vi "Module_Configure_All SMUs_Manual.vi"(7 "Throw Settings":T4={"SMU Settings"={"CH"={"Voltage Limit"=1.0, "current limit"=0.01, "Voltage limit range"=6.0, "Current level"=0.01, "CH_RF1"="0", "Output Enabled"=TRUE}, "CH"={"Voltage Limit"=1.0, "current limit"=0.01, "Voltage limit range"=6.0, "Current level"=0.01, "CH_RF2"="1", "Output Enabled"=TRUE}, "CH"={"Voltage Limit"=1.0, "current limit"=0.01, "Voltage limit range"=6.0, "Current level"=0.01, "CH_RF3"="2", "Output Enabled"=TRUE}, "CH"={"Voltage Limit"=1.0, "current limit"=0.01, "Voltage limit range"=6.0, "Current level"=0.01, "CH_RF4"="3", "Output Enabled"=TRUE}}, "sense"=1008, "aperture time"=0.01666} {"aperture time" format="%.2p"; "sense" items=["Local"=1008, "Remote"=1009]; "SMU Settings"."CH"."Current level" format="%#.6p"; "SMU Settings"."CH"."Voltage limit range" format="%#.6p"; "SMU Settings"."CH"."current limit" format="%#.6p"; "SMU Settings"."CH"."Voltage Limit" format="%#.6p"; "SMU Settings"."CH"."Current level" format="%#.6p"; "SMU Settings"."CH"."Voltage limit range" format="%#.6p"; "SMU Settings"."CH"."current limit" format="%#.6p"; "SMU Settings"."CH"."Voltage Limit" format="%#.6p"; "SMU Settings"."CH"."Current level" format="%#.6p"; "SMU Settings"."CH"."Voltage limit range" format="%#.6p"; "SMU Settings"."CH"."current limit" format="%#.6p"; "SMU Settings"."CH"."Voltage Limit" format="%#.6p"; "SMU Settings"."CH"."Current level" format="%#.6p"; "SMU Settings"."CH"."Voltage limit range" format="%#.6p"; "SMU Settings"."CH"."current limit" format="%#.6p"; "SMU Settings"."CH"."Voltage Limit" format="%#.6p"}, 8 "Error In":errorcluster, 10 "DUT and Bridge SMU Settings":T5={"SMU Settings"={"CH"={"voltage level range"=6.0, "current limit"=0.1, "current limit range"=0.1, "voltage level "=1.2, "CH"="0", "Output Enabled"=FALSE}, "CH 2"={"voltage level range"=6.0, "current limit"=0.001, "current limit range"=0.001, "voltage level "=5.0, "CH"="1", "Output Enabled"=FALSE}, "CH 3"={"voltage level range"=6.0, "current limit"=0.001, "current limit range"=0.001, "voltage level "=-5.0, "CH"="2", "Output Enabled"=FALSE}, "CH 4"={"voltage level range"=6.0, "current limit"=0.01, "current limit range"=0.01, "voltage level "=1.8, "CH"="3", "Output Enabled"=FALSE}}, "sense"=1008, "aperture time"=0.01666} {"aperture time" format="%.2p"; "sense" items=["Local"=1008, "Remote"=1009]; "SMU Settings"."CH 4"."voltage level" format="%#.6p"; "SMU Settings"."CH 4"."current limit range" format="%#.6p"; "SMU Settings"."CH 4"."current limit" format="%#.6p"; "SMU Settings"."CH 4"."voltage level range" format="%#.6p"; "SMU Settings"."CH 3"."voltage level" format="%#.6p"; "SMU Settings"."CH 3"."current limit range" format="%#.6p"; "SMU Settings"."CH 3"."current limit" format="%#.6p"; "SMU Settings"."CH 3"."voltage level range" format="%#.6p"; "SMU Settings"."CH 2"."voltage level" format="%#.6p"; "SMU Settings"."CH 2"."current limit range" format="%#.6p"; "SMU Settings"."CH 2"."current limit" format="%#.6p"; "SMU Settings"."CH 2"."voltage level range" format="%#.6p"; "SMU Settings"."CH"."voltage level" format="%#.6p"; "SMU Settings"."CH"."current limit range" format="%#.6p"; "SMU Settings"."CH"."current limit" format="%#.6p"; "SMU Settings"."CH"."voltage level range" format="%#.6p"}, 11 "Instrument_Visas":T1) -> (0 "Error Out":errorcluster, 2 "DUR_4_CH_SMU":T3(array[cluster]) {"sense 2" items=["Local"=1008, "Remote"=1009]}, 3 "Throw_4_CH_SMU":T3(array[cluster]) {"sense 2" items=["Local"=1008, "Remote"=1009]})   [LabVIEW 2013]
uses:
  <instrlib>/niDCPower/nidcpower.llb/niDCPower Sense.ctl
  <instrlib>/niDCPower/nidcpower.llb/niDCPower Aperture Time Units.ctl
  <instrlib>/niDCPower/nidcpower.llb/niDCPower Output Function.ctl
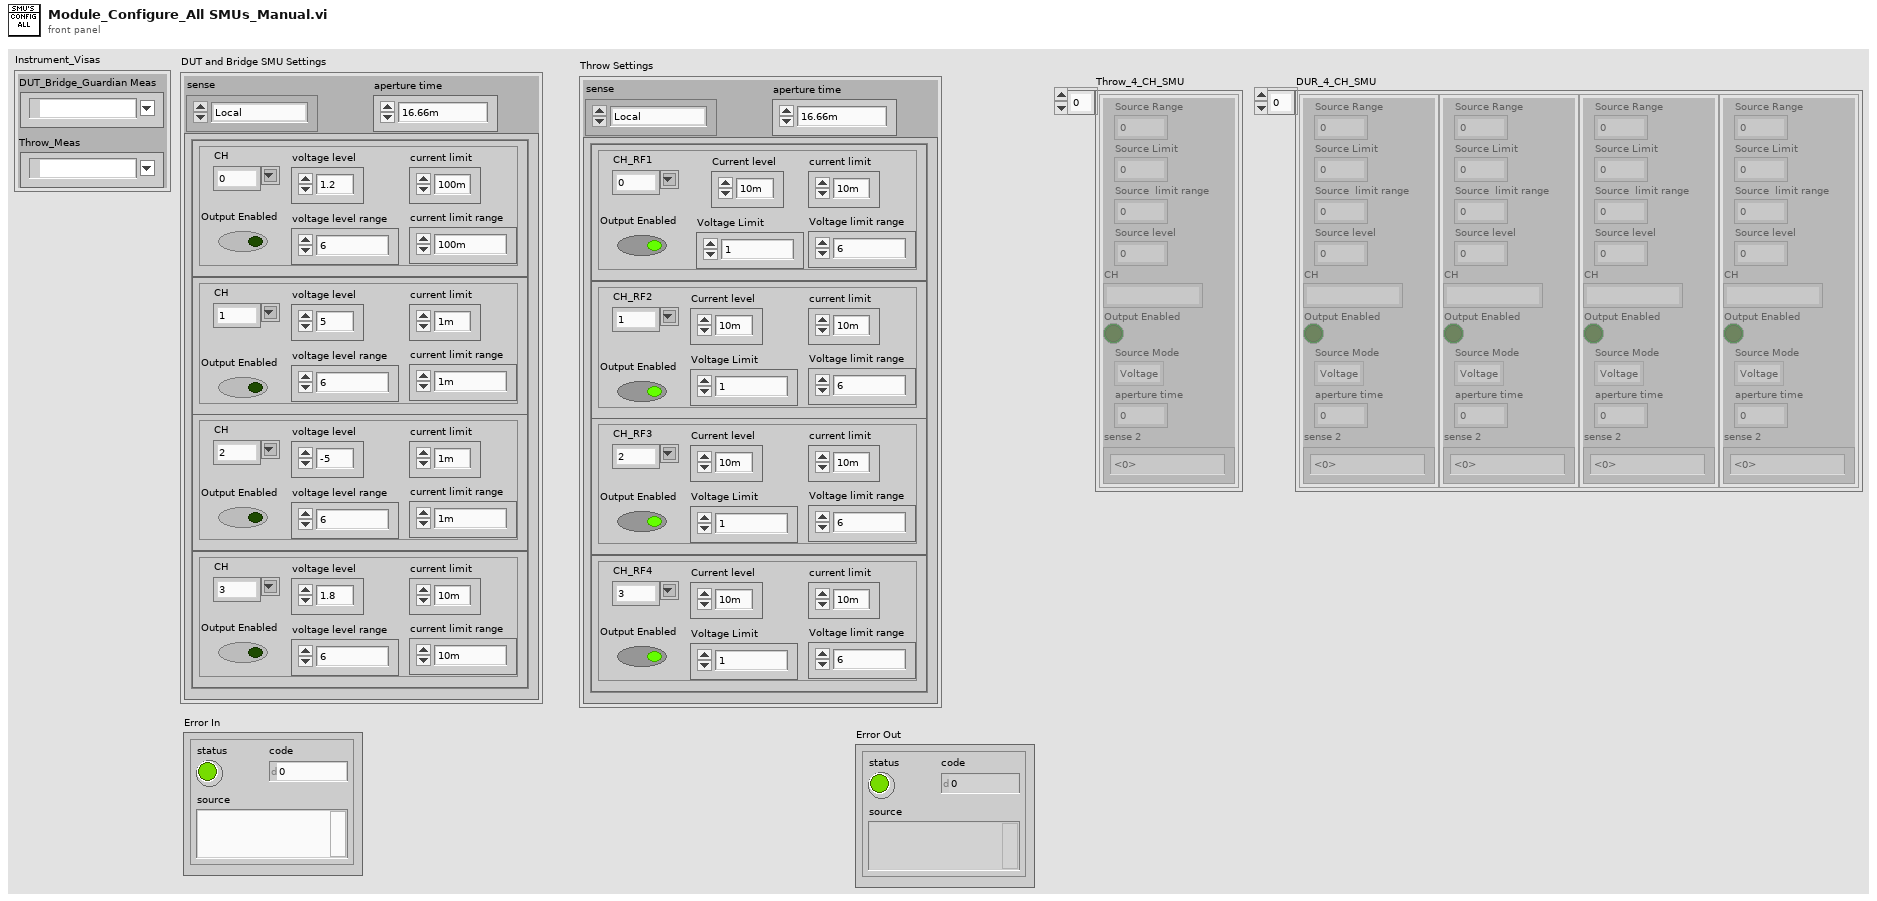
[diagram p1: front panel]
types:
  T1 = cluster{"DUT_Bridge_Guardian Meas":refnum<k15>, "Throw_Meas":refnum<k15>}
  T2 = typedef "niDCPower Sense.ctl" = i32
  T3 = cluster{"Source Range":dbl, "Source Limit":dbl, "Source  limit range":dbl, "Source level":dbl, "CH":string, "Output Enabled":bool, "Source Mode":enum16{"Voltage", "Current"}, "aperture time":dbl, "sense 2":T2}[]
  T4 = cluster{"SMU Settings":cluster{"CH":cluster{"Voltage Limit":dbl, "current limit":dbl, "Voltage limit range":dbl, "Current level":dbl, "CH_RF1":string, "Output Enabled":bool}, "CH":cluster{"Voltage Limit":dbl, "current limit":dbl, "Voltage limit range":dbl, "Current level":dbl, "CH_RF2":string, "Output Enabled":bool}, "CH":cluster{"Voltage Limit":dbl, "current limit":dbl, "Voltage limit range":dbl, "Current level":dbl, "CH_RF3":string, "Output Enabled":bool}, "CH":cluster{"Voltage Limit":dbl, "current limit":dbl, "Voltage limit range":dbl, "Current level":dbl, "CH_RF4":string, "Output Enabled":bool}}, "sense":T2, "aperture time":dbl}
  T5 = cluster{"SMU Settings":cluster{"CH":cluster{"voltage level range":dbl, "current limit":dbl, "current limit range":dbl, "voltage level ":dbl, "CH":string, "Output Enabled":bool}, "CH 2":cluster{"voltage level range":dbl, "current limit":dbl, "current limit range":dbl, "voltage level ":dbl, "CH":string, "Output Enabled":bool}, "CH 3":cluster{"voltage level range":dbl, "current limit":dbl, "current limit range":dbl, "voltage level ":dbl, "CH":string, "Output Enabled":bool}, "CH 4":cluster{"voltage level range":dbl, "current limit":dbl, "current limit range":dbl, "voltage level ":dbl, "CH":string, "Output Enabled":bool}}, "sense":T2, "aperture time":dbl}
  T6 = cluster{"CH":cluster{"voltage level range":dbl, "current limit":dbl, "current limit range":dbl, "voltage level ":dbl, "CH":string, "Output Enabled":bool}, "CH 2":cluster{"voltage level range":dbl, "current limit":dbl, "current limit range":dbl, "voltage level ":dbl, "CH":string, "Output Enabled":bool}, "CH 3":cluster{"voltage level range":dbl, "current limit":dbl, "current limit range":dbl, "voltage level ":dbl, "CH":string, "Output Enabled":bool}, "CH 4":cluster{"voltage level range":dbl, "current limit":dbl, "current limit range":dbl, "voltage level ":dbl, "CH":string, "Output Enabled":bool}}
  T7 = cluster{"voltage level range":dbl, "current limit":dbl, "current limit range":dbl, "voltage level ":dbl, "CH":string, "Output Enabled":bool}[]
  T8 = cluster{"Source Range":dbl, "Source Limit":dbl, "Source  limit range":dbl, "Source level":dbl, "CH":string, "Output Enabled":bool, "Source Mode":enum16{"Voltage", "Current"}, "aperture time":dbl, "sense 2":T2}
  T9 = typedef "niDCPower Output Function.ctl" = i32
  T10 = typedef "niDCPower Aperture Time Units.ctl" = i32
  T11 = cluster{"CH":cluster{"Voltage Limit":dbl, "current limit":dbl, "Voltage limit range":dbl, "Current level":dbl, "CH_RF1":string, "Output Enabled":bool}, "CH":cluster{"Voltage Limit":dbl, "current limit":dbl, "Voltage limit range":dbl, "Current level":dbl, "CH_RF2":string, "Output Enabled":bool}, "CH":cluster{"Voltage Limit":dbl, "current limit":dbl, "Voltage limit range":dbl, "Current level":dbl, "CH_RF3":string, "Output Enabled":bool}, "CH":cluster{"Voltage Limit":dbl, "current limit":dbl, "Voltage limit range":dbl, "Current level":dbl, "CH_RF4":string, "Output Enabled":bool}}
  T12 = cluster{"Voltage Limit":dbl, "current limit":dbl, "Voltage limit range":dbl, "Current level":dbl, "CH_RF4":string, "Output Enabled":bool}[]
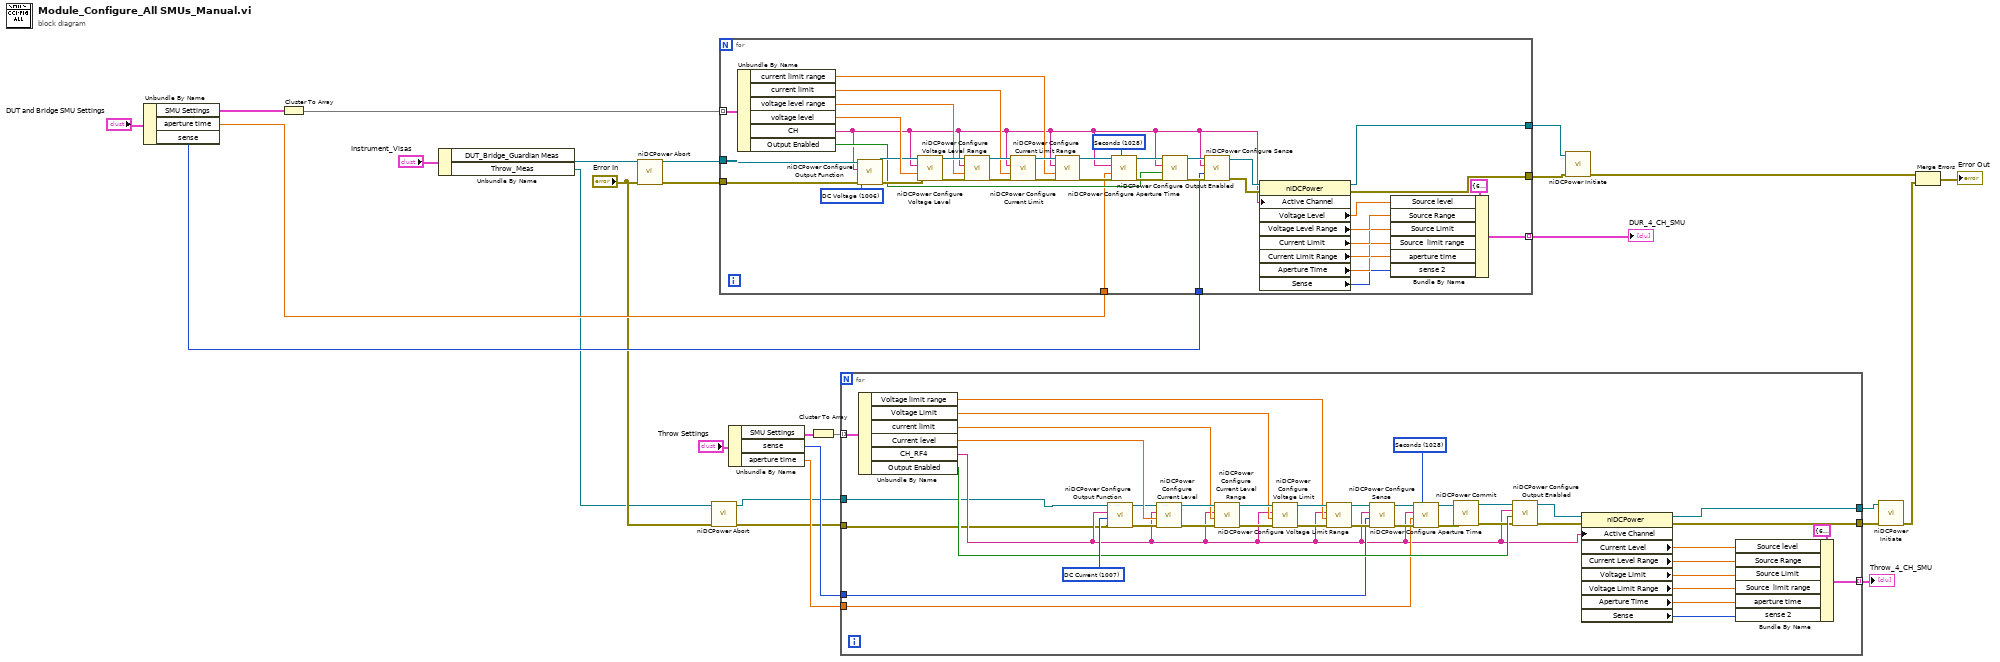
[diagram p0: block diagram]
diagram:
  n1 = Unbundle By Name("DUT and Bridge SMU Settings") -> ("SMU Settings"=w20:T6, "aperture time"=w23:dbl, "sense"=w22:T2)
  n2 = Cluster To Array(cluster=w20) -> (array=w12:T7)
  n3 = Unbundle By Name("Instrument_Visas") -> ("DUT_Bridge_Guardian Meas"=w25:refnum<k15>, "Throw_Meas"=w4:refnum<k15>)
  n4 = call <instrlib>:"niDCPower Abort.vi"("error in (no error)"="Error In", "instrument handle"=w25) -> ("error out"=w26:errorcluster, "instrument handle out"=w27:refnum<k15>)  [unwired: 8 in]
  n5 = call <instrlib>:"niDCPower Abort.vi"("error in (no error)"="Error In", "instrument handle"=w4) -> ("error out"=w6:errorcluster, "instrument handle out"=w5:refnum<k15>)  [unwired: 8 in]
  n6 = for {
    tunnel: w12 -> [w60] mode=indexing
    tunnel: w27 -> [w46]
    tunnel: [w29] -> w9
    tunnel: w26 -> [w44]
    tunnel: w23 -> [w42]
    tunnel: w22 -> [w41]
    tunnel: [w32] -> w21 mode=indexing
    tunnel: [w28] -> w10
    w48 = T9 1006 items=["DC Voltage"=1006, "DC Current"=1007, "Pulse Voltage"=1049, "Pulse Current"=1050] ("output function")
    w49 = T10 1028 items=["Seconds"=1028, "Powerline Cycles"=1029] ("aperture time units")
    n7 = Unbundle By Name(w60) -> ("current limit range"=w56:dbl, "current limit"=w57:dbl, "voltage level range"=w58:dbl, "voltage level"=w59:dbl, "CH"=w30:string, "Output Enabled"=w43:bool)
    n8 = call <instrlib>:"niDCPower Configure Output Function.vi"("error in (no error)"=w44, "output function"=w48, "channel name"=w30, "instrument handle"=w46) -> ("error out"=w47:errorcluster, "instrument handle out"=w45:refnum<k15>)  [unwired: 6 in]
    n9 = call <instrlib>:"niDCPower Configure Voltage Level.vi"("error in (no error)"=w47, "voltage level"=w59, "channel name"=w30, "instrument handle"=w45) -> ("error out"=w65:errorcluster, "instrument handle out"=w66:refnum<k15>)  [unwired: 6 in]
    n10 = call <instrlib>:"niDCPower Configure Voltage Level Range.vi"("error in (no error)"=w65, "voltage level range"=w58, "channel name"=w30, "instrument handle"=w66) -> ("error out"=w64:errorcluster, "instrument handle out"=w63:refnum<k15>)  [unwired: 6 in]
    n11 = call <instrlib>:"niDCPower Configure Current Limit.vi"("error in (no error)"=w64, "current limit"=w57, "channel name"=w30, "instrument handle"=w63) -> ("error out"=w62:errorcluster, "instrument handle out"=w61:refnum<k15>)  [unwired: 6 in]
    n12 = call <instrlib>:"niDCPower Configure Current Limit Range.vi"("error in (no error)"=w62, "current limit range"=w56, "channel name"=w30, "instrument handle"=w61) -> ("error out"=w53:errorcluster, "instrument handle out"=w50:refnum<k15>)  [unwired: 6 in]
    n13 = call <instrlib>:"niDCPower Configure Aperture Time.vi"("aperture time units"=w49, "error in (no error)"=w53, "aperture time"=w42, "channel name"=w30, "instrument handle"=w50) -> ("error out"=w52:errorcluster, "instrument handle out"=w51:refnum<k15>)  [unwired: 5 in]
    n14 = call <instrlib>:"niDCPower Configure Output Enabled.vi"("error in (no error)"=w52, "output enabled"=w43, "channel name"=w30, "instrument handle"=w51) -> ("error out"=w55:errorcluster, "instrument handle out"=w54:refnum<k15>)  [unwired: 6 in]
    n15 = call <instrlib>:"niDCPower Configure Sense.vi"("error in (no error)"=w55, "sense"=w41, "channel name"=w30, "instrument handle"=w54) -> ("error out"=w40:errorcluster, "instrument handle out"=w39:refnum<k15>)  [unwired: 6 in]
    n16 = property class="niDCPower"(reference=w39, error in=w40, "Active Channel"=w30) -> (reference out=w29:refnum<k15>, error out=w28:errorcluster, "Voltage Level"=w31:dbl, "Voltage Level Range"=w37:dbl, "Current Limit"=w36:dbl, "Current Limit Range"=w35:dbl, "Aperture Time"=w34:dbl, "Sense"=w33:i32)
    n17 = Bundle By Name(cluster=T8 {"Source Range"=6.0, "Source Limit"=0.01, "Source  limit range"=0.01, "Source level"=1.2, "CH"="0", "Output Enabled"=FALSE, "Source Mode"=enum."Voltage", "aperture time"=0.01666, "sense 2"=1009} ("CH 3"), "Source level"=w31, "Source Range"=w37, "Source Limit"=w36, "Source  limit range"=w35, "aperture time"=w34, "sense 2"=w33) -> (w32:T8)
  }
  "DUR_4_CH_SMU" <- w21
  n18 = Unbundle By Name("Throw Settings") -> ("SMU Settings"=w18:T11, "sense"=w16:T2, "aperture time"=w15:dbl)
  n19 = Cluster To Array(cluster=w18) -> (array=w17:T12)
  n20 = for {
    tunnel: w17 -> [w106] mode=indexing
    tunnel: w16 -> [w82]
    tunnel: w15 -> [w81]
    tunnel: [w71] -> w14 mode=indexing
    tunnel: [w68] -> w3
    tunnel: w6 -> [w69]
    tunnel: w5 -> [w70]
    tunnel: [w67] -> w2
    w105 = T9 1007 items=["DC Voltage"=1006, "DC Current"=1007, "Pulse Voltage"=1049, "Pulse Current"=1050] ("output function")
    w107 = T10 1028 items=["Seconds"=1028, "Powerline Cycles"=1029] ("aperture time units")
    n21 = Unbundle By Name(w106) -> ("Voltage limit range"=w83:dbl, "Voltage Limit"=w84:dbl, "current limit"=w85:dbl, "Current level"=w103:dbl, "CH_RF4"=w79:string, "Output Enabled"=w104:bool)
    n22 = call <instrlib>:"niDCPower Configure Output Function.vi"("error in (no error)"=w69, "output function"=w105, "channel name"=w79, "instrument handle"=w70) -> ("error out"=w89:errorcluster, "instrument handle out"=w92:refnum<k15>)  [unwired: 6 in]
    n23 = call <instrlib>:"niDCPower Configure Current Level.vi"("error in (no error)"=w89, "current level"=w103, "channel name"=w79, "instrument handle"=w92) -> ("error out"=w102:errorcluster, "instrument handle out"=w101:refnum<k15>)  [unwired: 6 in]
    n24 = call <instrlib>:"niDCPower Configure Current Level Range.vi"("error in (no error)"=w102, "current level range"=w85, "channel name"=w79, "instrument handle"=w101) -> ("error out"=w100:errorcluster, "instrument handle out"=w99:refnum<k15>)  [unwired: 6 in]
    n25 = call <instrlib>:"niDCPower Configure Voltage Limit.vi"("error in (no error)"=w100, "voltage limit"=w84, "channel name"=w79, "instrument handle"=w99) -> ("error out"=w98:errorcluster, "instrument handle out"=w97:refnum<k15>)  [unwired: 6 in]
    n26 = call <instrlib>:"niDCPower Configure Voltage Limit Range.vi"("error in (no error)"=w98, "voltage limit range"=w83, "channel name"=w79, "instrument handle"=w97) -> ("error out"=w96:errorcluster, "instrument handle out"=w95:refnum<k15>)  [unwired: 6 in]
    n27 = call <instrlib>:"niDCPower Configure Sense.vi"("error in (no error)"=w96, "sense"=w82, "channel name"=w79, "instrument handle"=w95) -> ("error out"=w94:errorcluster, "instrument handle out"=w93:refnum<k15>)  [unwired: 6 in]
    n28 = call <instrlib>:"niDCPower Configure Aperture Time.vi"("aperture time units"=w107, "error in (no error)"=w94, "aperture time"=w81, "channel name"=w79, "instrument handle"=w93) -> ("error out"=w91:errorcluster, "instrument handle out"=w90:refnum<k15>)  [unwired: 5 in]
    n29 = call <instrlib>:"niDCPower Commit.vi"("error in (no error)"=w91, "instrument handle"=w90) -> ("error out"=w88:errorcluster, "instrument handle out"=w86:refnum<k15>)  [unwired: 8 in]
    n30 = call <instrlib>:"niDCPower Configure Output Enabled.vi"("error in (no error)"=w88, "output enabled"=w104, "channel name"=w79, "instrument handle"=w86) -> ("error out"=w87:errorcluster, "instrument handle out"=w80:refnum<k15>)  [unwired: 6 in]
    n31 = property class="niDCPower"(reference=w80, error in=w87, "Active Channel"=w79) -> (reference out=w67:refnum<k15>, error out=w68:errorcluster, "Current Level"=w76:dbl, "Current Level Range"=w75:dbl, "Voltage Limit"=w74:dbl, "Voltage Limit Range"=w73:dbl, "Aperture Time"=w77:dbl, "Sense"=w78:i32)
    n32 = Bundle By Name(cluster=T8 {"Source Range"=6.0, "Source Limit"=0.01, "Source  limit range"=0.01, "Source level"=1.2, "CH"="0", "Output Enabled"=FALSE, "Source Mode"=enum."Voltage", "aperture time"=0.01666, "sense 2"=1009} ("CH 3"), "Source level"=w76, "Source Range"=w75, "Source Limit"=w74, "Source  limit range"=w73, "aperture time"=w77, "sense 2"=w78) -> (w71:T8)
  }
  "Throw_4_CH_SMU" <- w14
  n33 = call <instrlib>:"niDCPower Initiate.vi"("error in (no error)"=w10, "instrument handle"=w9) -> ("error out"=w8:errorcluster)  [unwired: 8 in, 1 out]
  n34 = call <instrlib>:"niDCPower Initiate.vi"("error in (no error)"=w3, "instrument handle"=w2) -> ("error out"=w1:errorcluster)  [unwired: 8 in, 1 out]
  n35 = Merge Errors(w8, w1) -> (→"Error Out":errorcluster)
